vi "Stop Actor.vi"(8 "error in (no error)":errorcluster, 9 "Emergency? (f)":bool, 10 "Actor ID":string, 11 "Actor Monitor in":refnum<class "Actor Monitor.lvclass">) -> (0 "error out":errorcluster, 3 "Actor Monitor out":refnum<class "Actor Monitor.lvclass">)   [LabVIEW 2018, in "Monitored Actor.lvlib" / "Actor Monitor.lvclass"]
doc: "Sends a stop or emergency stop message to the actor\n\nCopyright: MGI\nAuthored by: Derek Trepanier"
uses:
  Actor Monitor.lvclass
  <vilib>/ActorFramework/Message Enqueuer/Message Enqueuer.lvclass/Message Enqueuer.ctl
  <vilib>/ActorFramework/Stop Msg/Stop Msg.lvclass/Stop Msg.ctl
  <vilib>/ActorFramework/Message Enqueuer/Enqueue.vi
  <vilib>/ActorFramework/Message Enqueuer/Enqueue Critical.vi
  <vilib>/ActorFramework/Stop Msg/Stop Msg.lvclass
  C:/Program Files (x86)/National Instruments/LabVIEW 2018/vi.lib/ActorFramework/Message/Message.lvclass
  <vilib>/ActorFramework/Message Priority Queue/Priority Enqueue.vi
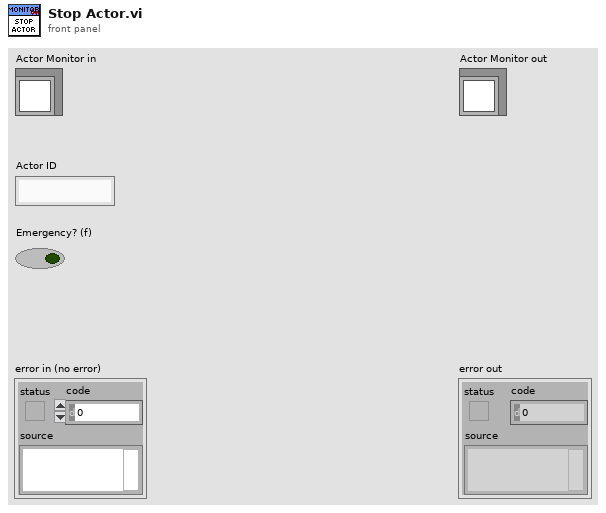
[diagram p1: front panel]
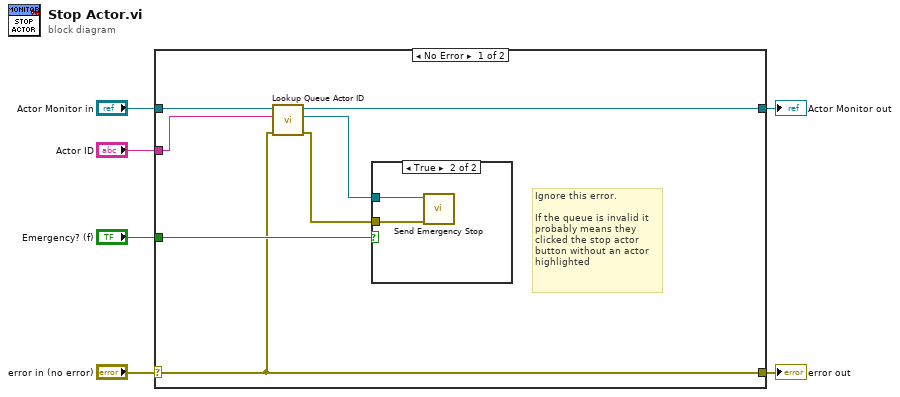
[diagram p0: block diagram]
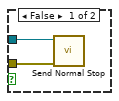
[diagram p2: hidden frame]
diagram:
  n1 = case shown="No Error" "error in (no error)" {
    selector: "error in (no error)" -> [w7 w19]
    tunnel: [w7 w19] -> w5
    tunnel: [w12 w18] -> w3
    tunnel: "Actor Monitor in" -> [w13 w18]
    tunnel: "Emergency? (f)" -> [w11 _]
    tunnel: "Actor ID" -> [w10 _]
    frame No Error {
      # "Ignore this error.\n\nIf the queue is invalid it probably means they clicked the stop actor button without an actor highlighted"
      n2 = call "Lookup Queue Actor ID.vi"("error in (no error)"=w7, "Actor ID"=w10, "Actor Monitor in"=w13) -> ("error out"=w9:errorcluster, "Actor's Queue"=w8:refnum<class "Message Enqueuer.lvclass">, "Actor Monitor out"=w12:refnum<class "Actor Monitor.lvclass">)  [unwired: 6 in]
      n3 = case shown="True" w11 {
        tunnel: w9 -> [w14 w17]
        tunnel: w8 -> [w15 w16]
        frame False {
          n4 = call <vilib>:"Send Normal Stop.vi"("error in (no error)"=w14, "Message Enqueuer"=w15) -> ()  [unwired: 9 in, 1 out]
        }
        frame True {
          n5 = call <vilib>:"Send Emergency Stop.vi"("error in (no error)"=w17, "Message Enqueuer"=w16) -> ()  [unwired: 9 in, 1 out]
        }
      }
    }
    frame Error {
    }
  }
  "error out" <- w5
  "Actor Monitor out" <- w3
